vi "0_Dataset_Aug.vi"() -> ()   [LabVIEW 2020]
uses:
  Controls/Aug_Flip.ctl
  <vilib>/vision/NI_Vision_Development_Module.lvlib
panel:
  out "Annotations without images":path[](array[path])
  in  "Destinsation Path (Images)":path=path "D:/Ngene/GitHub/deepltk_examples/3_Image_Processing/33_Object_Detection/Dataset/1_Aug(4x)/Train/Images"
  out "Images without Annotation":path[](array[path])=[path "D:/Ngene/GitHub/deepltk_examples/3_Image_Processing/33_Object_Detection/Dataset/Orig/Train/Images/461.png", path "D:/Ngene/GitHub/deepltk_examples/3_Image_Processing/33_Object_Detection/Dataset/Orig/Train/Images/462.png", path "D:/Ngene/GitHub/deepltk_examples/3_Image_Processing/33_Object_Detection/Dataset/Orig/Train/Images/463.png", path "D:/Ngene/GitHub/deepltk_examples/3_Image_Processing/33_Object_Detection/Dataset/Orig/Train/Images/464.png", path "D:/Ngene/GitHub/deepltk_examples/3_Image_Processing/33_Object_Detection/Dataset/Orig/Train/Images/465.png", path "D:/Ngene/GitHub/deepltk_examples/3_Image_Processing/33_Object_Detection/Dataset/Orig/Train/Images/466.png", path "D:/Ngene/GitHub/deepltk_examples/3_Image_Processing/33_Object_Detection/Dataset/Orig/Train/Images/467.png", path "D:/Ngene/GitHub/deepltk_examples/3_Image_Processing/33_Object_Detection/Dataset/Orig/Train/Images/468.png", path "D:/Ngene/GitHub/deepltk_examples/3_Image_Processing/33_Object_Detection/Dataset/Orig/Train/Images/469.png", path "D:/Ngene/GitHub/deepltk_examples/3_Image_Processing/33_Object_Detection/Dataset/Orig/Train/Images/470.png", path "D:/Ngene/GitHub/deepltk_examples/3_Image_Processing/33_Object_Detection/Dataset/Orig/Train/Images/471.png", path "D:/Ngene/GitHub/deepltk_examples/3_Image_Processing/33_Object_Detection/Dataset/Orig/Train/Images/472.png", path "D:/Ngene/GitHub/deepltk_examples/3_Image_Processing/33_Object_Detection/Dataset/Orig/Train/Images/473.png", path "D:/Ngene/GitHub/deepltk_examples/3_Image_Processing/33_Object_Detection/Dataset/Orig/Train/Images/474.png", path "D:/Ngene/GitHub/deepltk_examples/3_Image_Processing/33_Object_Detection/Dataset/Orig/Train/Images/7.png"]
  in  "Image Quality":u32=1000 max=1000
  in  "Save Format":enum16{"JPEG", "PNG", "BMP"}(ring)
  in  "Destinsation Path (Annotations)":path=path "D:/Ngene/GitHub/deepltk_examples/3_Image_Processing/33_Object_Detection/Dataset/1_Aug(4x)/Train/Annotations"
  in  "Aug Factor":enum16{"2x", "4x", "8x"}(ring)=enum."4x"
  out "error out":errorcluster
  in  "Source Path (Annotations)":path=path "D:/Ngene/GitHub/deepltk_examples/3_Image_Processing/33_Object_Detection/Dataset/0_Orig/Train/Annotations"
  in  "Source Path (Images)":path=path "D:/Ngene/GitHub/deepltk_examples/3_Image_Processing/33_Object_Detection/Dataset/0_Orig/Train/Images"
  out "Total":i32=306
  out "Processed":i32=305
  # "Overview: This VI performs dataset augmentation by applyling flip and rotation transformations to images and associated BBox annotations if available. \nRequirements: \n1. Vision Development Module.\nInstructions:\n1. Provide the dataset paths to images and annotations(optional) at \"Dataset (Images)\" and \"Dataset (Annotations)\".\n2. Provide the destination paths for images and annotations at \"Images Destination\" and \"Annotation Destination\".\n3. Provide Augmentation factor:\n – 2X: Applies vertical flip only.\n – 4X: Applies vertical flip, rotation (180°), and flip + rotation (180°).\n – 8X: Applies all combinations of vertical flip, 90°, 180°, 270° rotations, and flip + rotate.\n4. Set saving format and quality for augmented images at \"Save Format\" and \"Image Quality\".\n5. Run the VI and wait until augmentation is done."
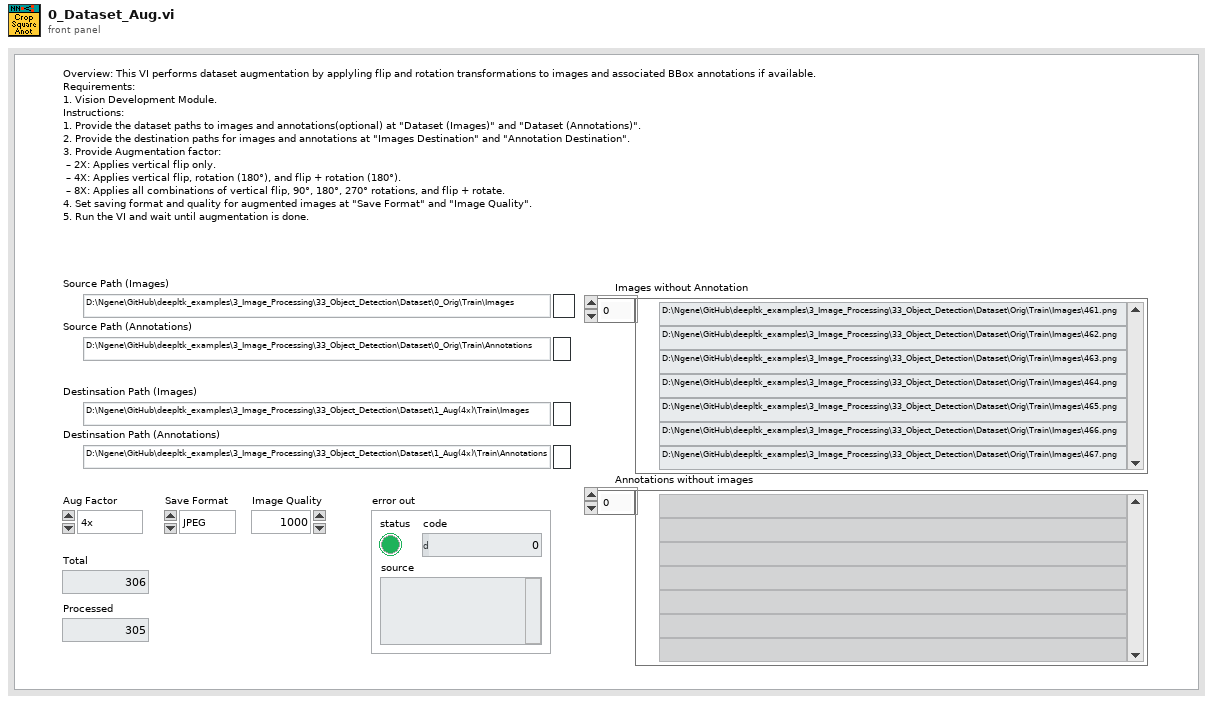
[diagram p1: front panel]
types:
  T1 = typedef "Image Type" = u32
  T2 = typedef "IMAQ Image.ctl" = refnum<image>
  T3 = typedef "Aug_Rotation.ctl" = enum16{"0", "90", "180", "270"}
  T4 = typedef "Aug_Flip.ctl" = enum16{"None", "Vertical", "Horizontal"}
  T5 = typedef "Deep_Learning_Toolkit_by_Ngene.lvlib/NN_BBox_Annotation.ctl" = cluster{"Class":i32, "BBox":T6}
  T6 = typedef "Deep_Learning_Toolkit_by_Ngene.lvlib/NN_BBox.ctl" = cluster{"x":sgl, "y":sgl, "w":sgl, "h":sgl}
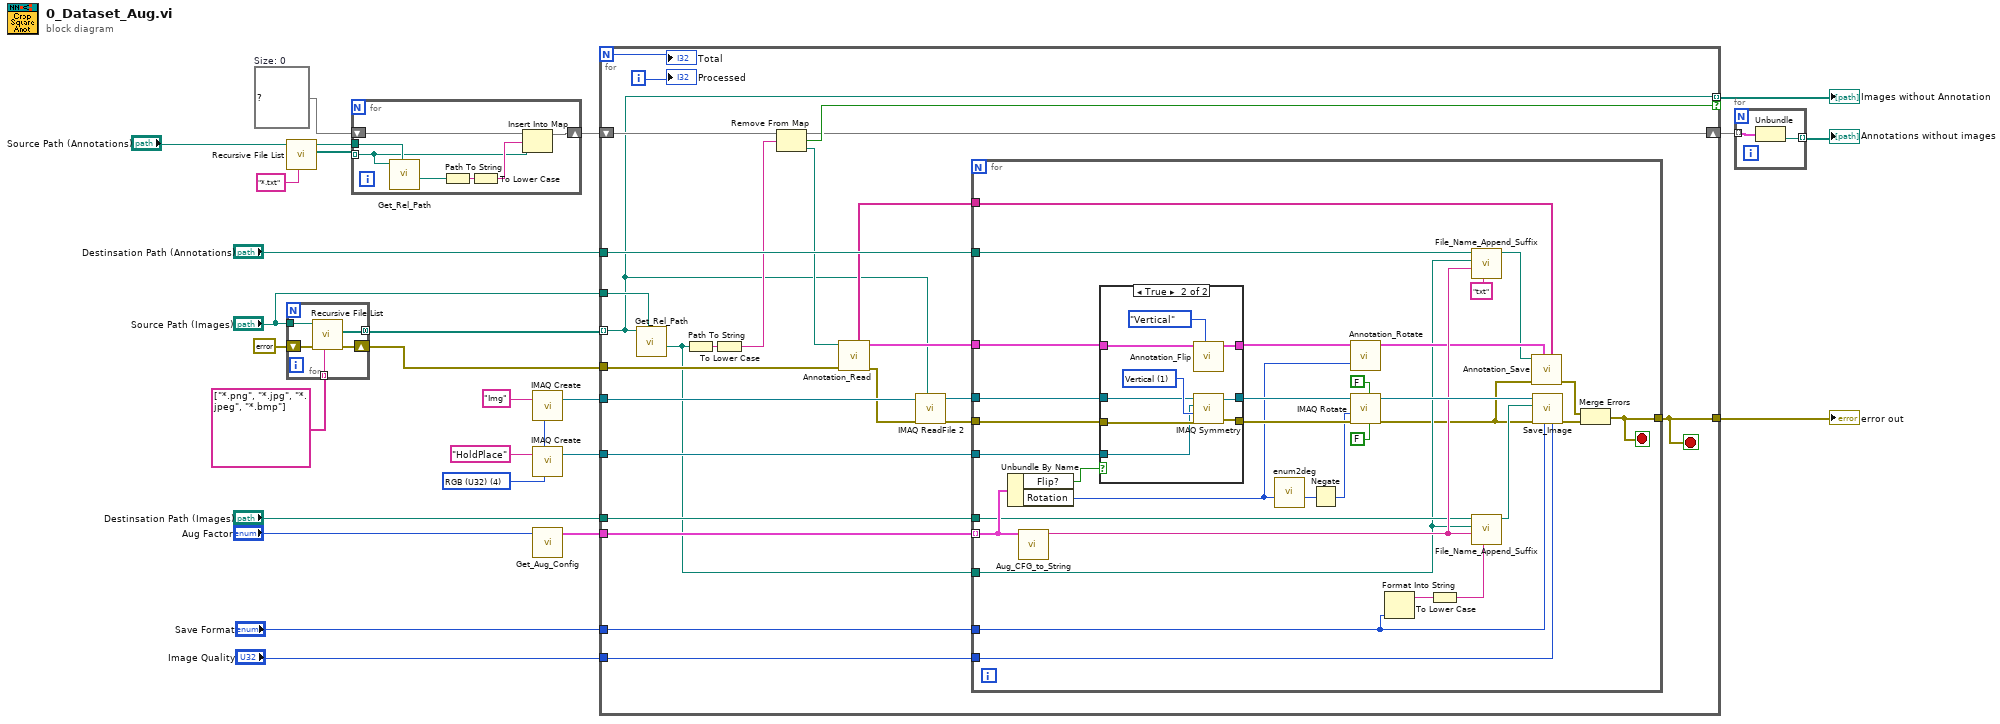
[diagram p0: block diagram]
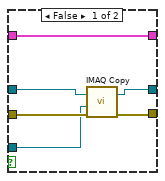
[diagram p2: hidden frame]
diagram:
  w4 = map{string, path} {}  # Size: 0
  w10 = T1 4 items=["Grayscale (U8)", "Grayscale (I16)", "Grayscale (SGL)", "Complex (CSG)", "RGB (U32)", "HSL (U32)", "RGB (U64)", "Grayscale (U16)"] ("Image Type")
  n1 = call <vilib>:"Recursive File List.vi"("pattern"="*.txt", "Folder Path"="Source Path (Annotations)") -> ("All Files in Dir"=w19:path[], "dup Folder Path"=w11:path)  [unwired: 5 in, 3 out]
  n2 = for {
    tunnel: "Source Path (Images)" -> [w31]
    tunnel: string[] ["*.png", "*.jpg", "*.jpeg", "*.bmp"] ("pattern") -> [w30] mode=indexing
    tunnel: [w29] -> w5 mode=concatenating
    shift-right: [w27] -> w2
    shift-left: errorcluster {"status"=FALSE, "code"=0, "source"=""} ("error out") -> [w28]
    n3 = call <vilib>:"Recursive File List.vi"("pattern"=w30, "error in (no error)"=w28, "Folder Path"=w31) -> ("error out"=w27:errorcluster, "All Files in Dir"=w29:path[])  [unwired: 4 in, 3 out]
  }
  n4 = for {
    tunnel: w19 -> [w32] mode=indexing
    shift-right: [w37] -> w18
    shift-left: w4 -> [w38]
    tunnel: w11 -> [w35]
    n5 = call "Get_Rel_Path.vi"("Parrent Folder"=w35, "Source File"=w32) -> ("Rel Path without extension"=w36:path)  [unwired: 6 in, 3 out]
    n6 = Path To String(path=w36) -> (string=w34:string)
    n7 = To Lower Case(string=w34) -> (all lower case string=w33:string)
    n8 = Insert Into Map(map in=w38, key=w33, value=w32) -> (map out=w37:map{string, path})  [unwired: 2 out]
  }
  n9 = call "IMAQ Create"("Image Name"="Img", "Image Type"=w10) -> ("New Image"=w23:T2)  [unwired: 3 in, 1 out]
  n10 = call "IMAQ Create"("Image Name"="HoldPlace", "Image Type"=w10) -> ("New Image"=w12:T2)  [unwired: 3 in, 1 out]
  n11 = call "Get_Aug_Config.vi"("Aug Factor"="Aug Factor") -> ("Aug_Config"=w20:cluster{"Flip?":bool, "Rotation":T3}[])  [unwired: 10 in]
  n12 = for {
    N -> [w63]
    tunnel: w2 -> [w60]
    tunnel: w23 -> [w61]
    tunnel: [w57] -> w22
    tunnel: w20 -> [w56]
    tunnel: "Destinsation Path (Annotations)" -> [w53]
    tunnel: "Save Format" -> [w52]
    tunnel: "Image Quality" -> [w51]
    tunnel: [w39] -> w15 mode=indexing if=w50
    tunnel: w12 -> [w49]
    tunnel: "Destinsation Path (Images)" -> [w46]
    shift-right: [w44] -> w8
    shift-left: w18 -> [w45]
    tunnel: "Source Path (Images)" -> [w43]
    tunnel: w5 -> [w39] mode=indexing
    i -> [w62]
    stop <- w57 stop-if-true
    n13 = call "Get_Rel_Path.vi"("Parrent Folder"=w43, "Source File"=w39) -> ("Rel Path without extension"=w40:path)  [unwired: 6 in, 3 out]
    n14 = Path To String(path=w40) -> (string=w42:string)
    n15 = To Lower Case(string=w42) -> (all lower case string=w41:string)
    n16 = Remove From Map(10:w41, 11:w45) -> (1:w48:path, 2:w50:bool, 3:w44:map{string, path})
    n17 = call "Annotation_Read.vi"("error in (no error)"=w60, "Path"=w48) -> ("error out"=w59:errorcluster, "Annotations (CWH)"=w58:T5[], "Class Names"=w47:string[])  [unwired: 7 in]
    n18 = call "IMAQ ReadFile 2"("File Path"=w39, "error in (no error)"=w59, "Image"=w61) -> ("error out"=w54:errorcluster, "Image Out"=w55:T2)  [unwired: 4 in, 3 out]
    n19 = for {
      tunnel: w55 -> [w94]
      tunnel: w47 -> [w93]
      tunnel: w58 -> [w95]
      tunnel: w54 -> [w92]
      tunnel: [w66] -> w57
      tunnel: w56 -> [w75] mode=indexing
      tunnel: w53 -> [w87]
      tunnel: w52 -> [w69]
      tunnel: w51 -> [w86]
      tunnel: w49 -> [w76]
      tunnel: w40 -> [w73]
      tunnel: w46 -> [w74]
      stop <- w66 stop-if-true
      n20 = Unbundle By Name(w75) -> ("Flip?"=w90:bool, "Rotation"=w64:T3)
      n21 = call "Aug_CFG_to_String.vi"("Config"=w75) -> ("Aug_Name"=w80:string)  [unwired: 10 in]
      n22 = case shown="True" w90 {
        tunnel: w95 -> [w100 w110]
        tunnel: w94 -> [w98 w107]
        tunnel: [w99 w106] -> w89
        tunnel: [w97 w105] -> w88
        tunnel: w92 -> [w101 w104]
        tunnel: [w100 w103] -> w91
        tunnel: w76 -> [w96 w102]
        frame False {
          n23 = call "IMAQ Copy"("error in (no error)"=w101, "Image Dst"=w96, "Image Src"=w98) -> ("error out"=w99:errorcluster, "Image Dst Out"=w97:T2)  [unwired: 3 in]
        }
        frame True {
          w108 = u32 1 items=["Horizontal", "Vertical", "Central", "1st Diagonal", "2nd Diagonal"] ("Type of Symmetry")
          n24 = call "Annotation_Flip.vi"("Flip"=Aug_Flip."Vertical", "Annotations (CWH)"=w110) -> ("Annotations (CWH) out"=w103:T5[])  [unwired: 9 in]
          n25 = call "IMAQ Symmetry"("error in (no error)"=w104, "Type of Symmetry"=w108, "Image Dst"=w102, "Image Src"=w107) -> ("error out"=w106:errorcluster, "Image Dst Out"=w105:T2)  [unwired: 1 in]
        }
      }
      n26 = call "enum2deg.vi"("Rotation"=w64) -> ("number"=w82:i32)  [unwired: 10 in]
      n27 = Negate(x=w82) -> (-x=w81:i32)
      n28 = call "Annotation_Rotate.vi"("Rotation"=w64, "Annotations (CWH)"=w91) -> ("Annotations (CWH) out"=w79:T5[])  [unwired: 9 in]
      n29 = call "IMAQ Rotate"("Use Bilinear Interpolation"=FALSE, "Maintain Size"=FALSE, "error in (no error)"=w89, "Angle (degrees)"=w81, "Image Src"=w88) -> ("error out"=w65:errorcluster, "Image Dst Out"=w84:T2)  [unwired: 5 in]
      n30 = Format Into String(w69) -> (resulting string=w72:string)  [unwired: 3 in, 1 out]
      n31 = To Lower Case(string=w72) -> (all lower case string=w71:string)
      n32 = call "File_Name_Append_Suffix.vi"("New File Extension"="txt", "Suffix"=w80, "Rel_Path"=w73, "Dest"=w87) -> ("Dest Path"=w78:path)  [unwired: 7 in]
      n33 = call "File_Name_Append_Suffix.vi"("New File Extension"=w71, "Suffix"=w80, "Rel_Path"=w73, "Dest"=w74) -> ("Dest Path"=w83:path)  [unwired: 7 in]
      n34 = call "Annotation_Save.vi"("Class Names"=w93, "Annotations (CWH)"=w79, "error in (no error)"=w65, "appended path"=w78) -> ("error out"=w67:errorcluster)  [unwired: 7 in]
      n35 = call "Save_Image.vi"("Image Quality"=w86, "Save Format"=w69, "error in (no error)"=w65, "Dest Path"=w83, "Refnum in"=w84) -> ("error out"=w68:errorcluster)  [unwired: 5 in, 1 out]
      n36 = Merge Errors(w67, w68) -> (w66:errorcluster)
    }
    "Total" <- w63
    "Processed" <- w62
  }
  "error out" <- w22
  "Images without Annotation" <- w15
  n37 = for {
    tunnel: w8 -> [w112] mode=indexing
    tunnel: [w111] -> w7 mode=indexing
    n38 = Unbundle(w112) -> (w111:path)  [unwired: 1 out]
  }
  "Annotations without images" <- w7
